vi "Tester 1.vi"() -> ()   [LabVIEW 2020]
panel:
  out "Object out":refnum<class>
  out "String out":string
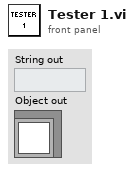
[diagram p1: front panel]
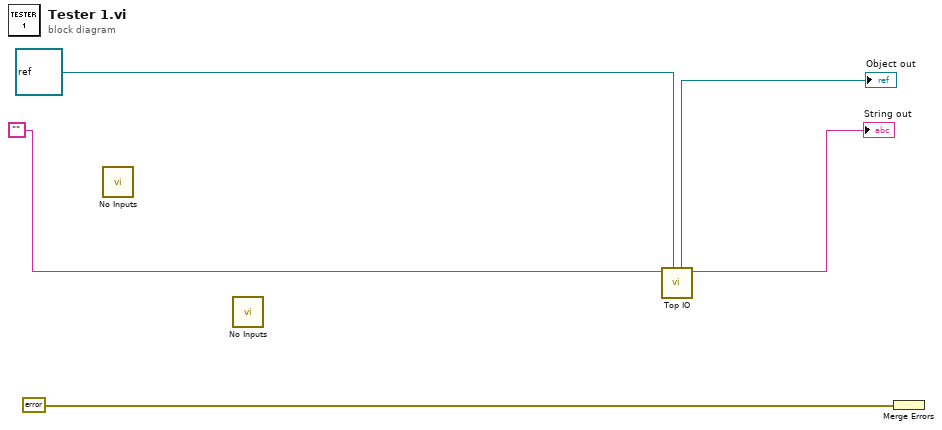
[diagram p0: block diagram]
diagram:
  n1 = call "No Inputs.vi"() -> ()  [unwired: 12 in]
  n2 = call "No Inputs.vi"() -> ()  [unwired: 12 in]
  n3 = call "Top IO.vi"("Object in"=refnum<class> refnum ("LabVIEW Object"), "String in"="") -> ("String out"=→"String out":string, "Object out"=→"Object out":refnum<class>)  [unwired: 8 in]
  n4 = Merge Errors(errorcluster {"status"=FALSE, "code"=0, "source"=""} ("error constant")) -> ()  [unwired: 1 out]
